vi "auto-optimize_grid-method.vi"() -> ()   [LabVIEW 2024]
panel:
  out "max indexes":i32[](array[numeric])
  out "yOut":dbl
  out "xOut":dbl
  out "max value":dbl
  out "Array":dbl[][](array[numeric])
  in  "start-y":dbl=75.0
  in  "start-x":dbl=75.0
  in  "auto-delta":dbl=0.5
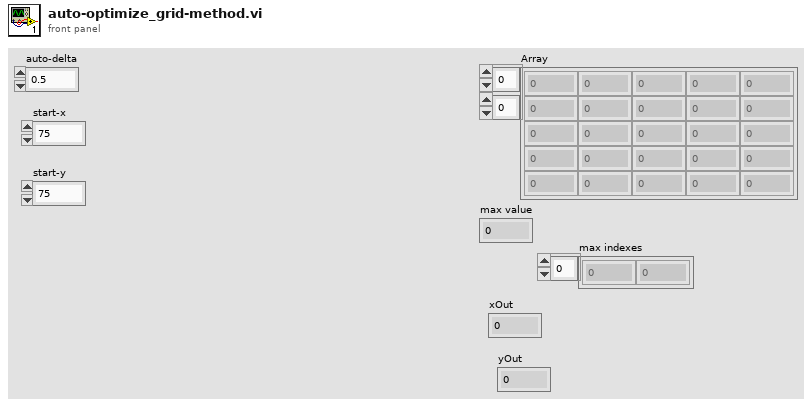
[diagram p1: front panel]
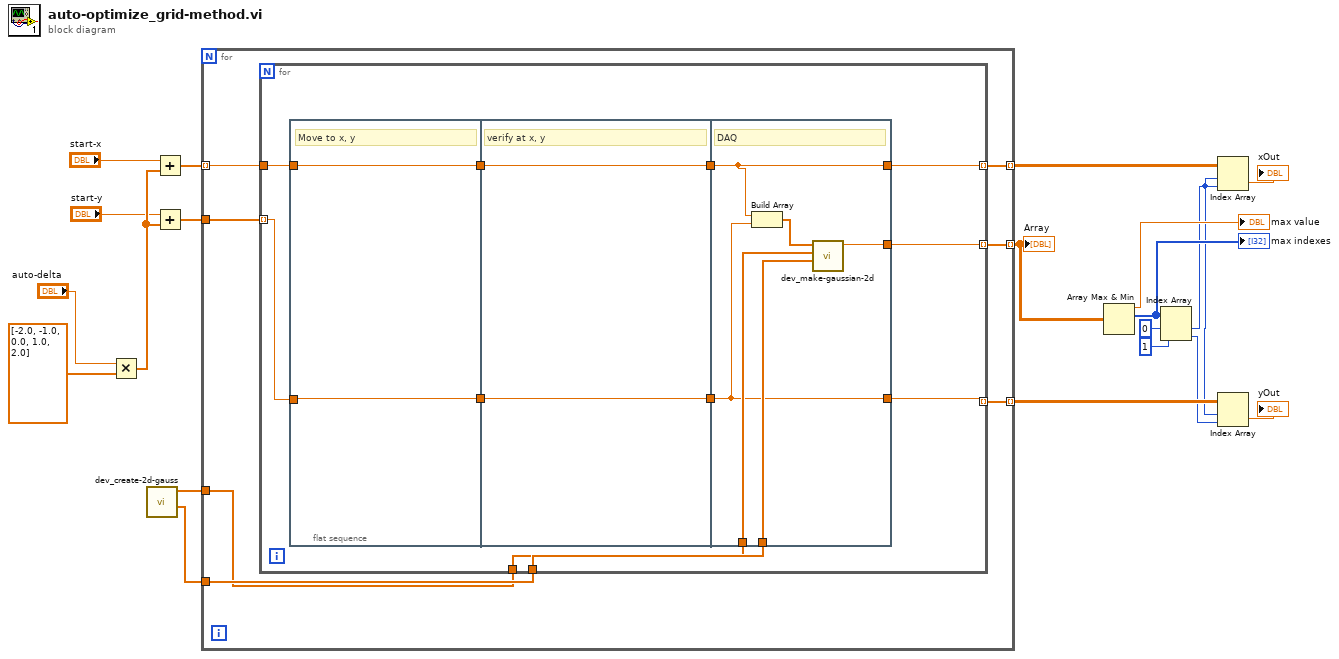
[diagram p0: block diagram]
diagram:
  n1 = Multiply(x="auto-delta", y=dbl[] [-2.0, -1.0, 0.0, 1.0, 2.0]) -> (x*y=w20:dbl[])
  n2 = call "dev_create-2d-gauss.vi"() -> ("StdDev"=w13:dbl[], "Mean"=w12:dbl[])  [unwired: 7 in, 3 out]
  n3 = Add(x="start-x", y=w20) -> (x+y=w17:dbl[])
  n4 = Add(x="start-y", y=w20) -> (x+y=w18:dbl[])
  n5 = for {
    tunnel: w17 -> [w26] mode=indexing
    tunnel: w18 -> [w27]
    tunnel: [w25] -> w6 mode=indexing
    tunnel: [w24] -> w4 mode=indexing
    tunnel: w13 -> [w23]
    tunnel: w12 -> [w22]
    tunnel: [w21] -> w11 mode=indexing
    n6 = for {
      tunnel: w27 -> [w38] mode=indexing
      tunnel: w26 -> [w37]
      tunnel: [w36] -> w24 mode=indexing
      tunnel: [w35] -> w25 mode=indexing
      tunnel: w23 -> [w34]
      tunnel: w22 -> [w33]
      tunnel: [w32] -> w21 mode=indexing
      n7 = flat-sequence {
        tunnel: w38 -> [w39]
        tunnel: w37 -> [w40]
        tunnel: [w40] -> w31
        tunnel: [w39] -> w29
        tunnel: w31 -> [w42]
        tunnel: [w42] -> w30
        tunnel: w29 -> [w41]
        tunnel: [w41] -> w28
        tunnel: [w46] -> w36
        tunnel: w30 -> [w46]
        tunnel: [w45] -> w35
        tunnel: w28 -> [w45]
        tunnel: w34 -> [w48]
        tunnel: w33 -> [w47]
        tunnel: [w43] -> w32
        frame #0 {
          # "Move to x, y"
        }
        frame #1 {
          # "verify at x, y"
        }
        frame #2 {
          # "DAQ"
          n8 = Build Array(w46, w45) -> (w44:dbl[])
          n9 = call "dev_make-gaussian-2d.vi"("StdDev"=w48, "Mean"=w47, "in"=w44) -> ("out"=w43:dbl)  [unwired: 8 in]
        }
      }
    }
  }
  "Array" <- w11
  n10 = Array Max & Min(array=w11) -> (max value=→"max value":dbl, max index (indices)=w9:i32[])  [unwired: 2 out]
  "max indexes" <- w9
  n11 = Index Array(array=w9, index #1=0 ("index"), index #2=1 ("index")) -> (element #1=w3:i32, element #2=w5:i32)
  n12 = Index Array(array=w4, index (row)=w3, index (col)=w3) -> (element=→"xOut":dbl)
  n13 = Index Array(array=w6, index (row)=w3, index (col)=w5) -> (element=→"yOut":dbl)
